vi "SUB_SFCS_GetUSNItem.vi"(0 "URL":string="10.41.21.182:136", 1 "SN":string="21GF0AA2IJ", 2 "Stage":string="AO", 3 "CATEGORY":string="51", 4 "SEQ":i32) -> (5 "Status":string)   [LabVIEW 2011]
uses:
  data/MCSDLL.dll
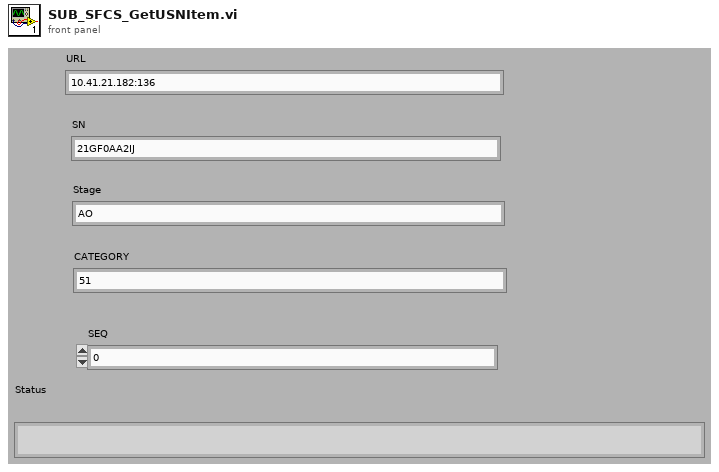
[diagram p1: front panel]
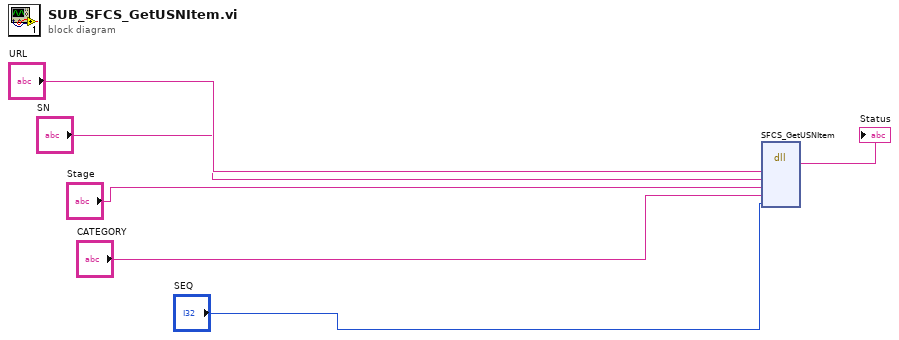
[diagram p0: block diagram]
diagram:
  n1 = dll-call lib="D:/S8300E_Project/data/MCSDLL.dll" fn="SFCS_GetUSNItem"("URL"="URL", "SN"="SN", "Stage"="Stage", "CATEGORY"="CATEGORY", "SEQ"="SEQ") -> (→"Status":string)  [unwired: 8 in, 2 out]
